vi "GenerateData.vi"(8 "error in (no error)":errorcluster, 11 "DemoStage in":refnum<class "DemoStage.lvclass">) -> (0 "error out":errorcluster, 2 "DataExchange":T1, 3 "DemoStage out":refnum<class "DemoStage.lvclass">)   [LabVIEW 2020, in "DemoStage.lvlib" / "DemoStage.lvclass"]
uses:
  DemoStage.lvclass
  Hardware Abstraction Layer/Component/Device/Device/DataExchange.ctl
  Hardware Abstraction Layer/Component/Stage/Stage/Stage.lvclass
  Interface/DataListener/DataListener.lvclass
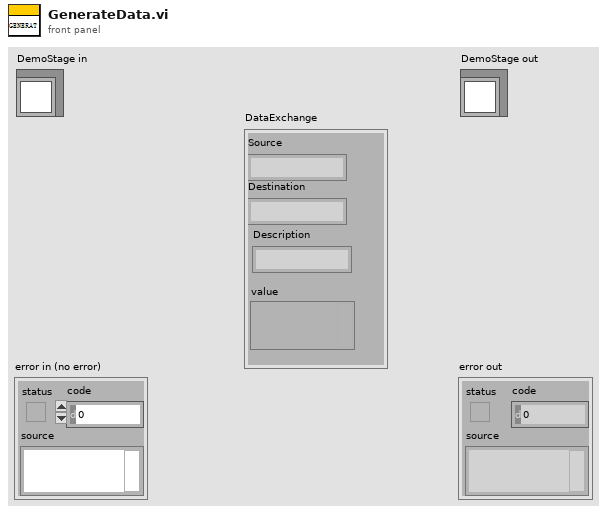
[diagram p1: front panel]
types:
  T1 = typedef "DataListener.lvclass/DataExchange.ctl" = cluster{"Source":string, "Destination":string, "Description":string, "value":variant}
  T2 = cluster{"Stage X Position":dbl, "Stage Y Position":dbl, "Stage Z Position":dbl}
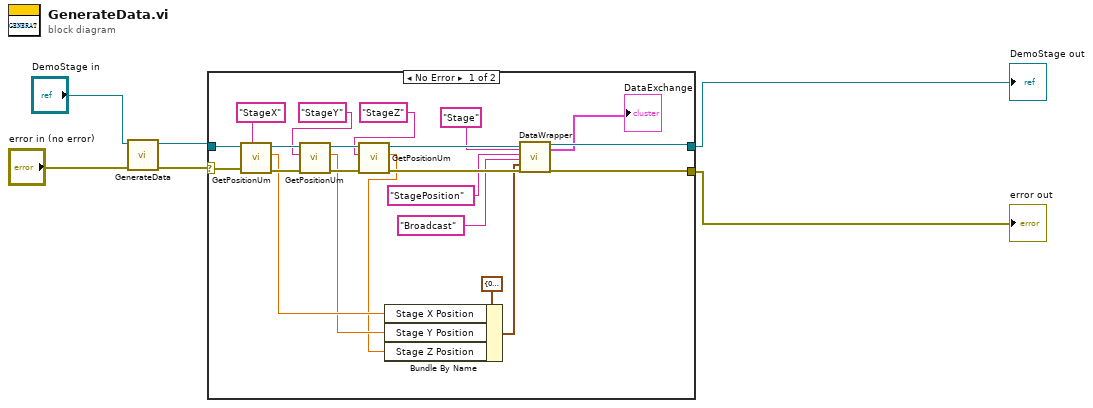
[diagram p0: block diagram]
diagram:
  n1 = call-parent "GenerateData.vi"("error in (no error)"="error in (no error)", "Device in"="DemoStage in") -> ("error out"=w3:errorcluster, "Device out"=w4:refnum<class "DemoStage.lvclass">)  [unwired: 7 in, 1 out]
  n2 = case shown="No Error" w3 {
    selector: w3 -> [w22 w30]
    tunnel: [w17 w30] -> w1
    tunnel: [w15 w29] -> w2
    tunnel: w4 -> [w28 w29]
    frame No Error {
      n3 = call-dynamic "GetPositionUm.vi"("error in (no error)"=w22, "Stage Label"="StageX", "DemoStage in"=w28) -> ("error out"=w21:errorcluster, "Stage Position"=w10:dbl, "DemoStage out"=w27:refnum<class "DemoStage.lvclass">)  [unwired: 6 in]
      n4 = call-dynamic "GetPositionUm.vi"("error in (no error)"=w21, "Stage Label"="StageY", "DemoStage in"=w27) -> ("error out"=w20:errorcluster, "Stage Position"=w9:dbl, "DemoStage out"=w26:refnum<class "DemoStage.lvclass">)  [unwired: 6 in]
      n5 = call-dynamic "GetPositionUm.vi"("error in (no error)"=w20, "Stage Label"="StageZ", "DemoStage in"=w26) -> ("error out"=w19:errorcluster, "Stage Position"=w8:dbl, "DemoStage out"=w16:refnum<class "DemoStage.lvclass">)  [unwired: 6 in]
      n6 = Bundle By Name(cluster=T2 {"Stage X Position"=0.0, "Stage Y Position"=0.0, "Stage Z Position"=0.0} ("Cluster"), "Stage X Position"=w10, "Stage Y Position"=w9, "Stage Z Position"=w8) -> (w14:T2)
      n7 = call-dynamic "DataWrapper.vi"("Device in"=w16, "Source"="Stage", "Description"="StagePosition" ("Target"), "Destination"="Broadcast" ("Type"), "value"=w14, "error in (no error)"=w19) -> ("Device out"=w15:refnum<class "DemoStage.lvclass">, "DataExchange"=→"DataExchange":T1, "error out"=w17:errorcluster)  [unwired: 11 in]
    }
    frame Error {
    }
  }
  "error out" <- w1
  "DemoStage out" <- w2
